vi "FTW-Supervisor-Core-Process.vi"(0 "FTW Supervisor Configuration":string, 11 "error in":errorcluster) -> (15 "error out":errorcluster)   [LabVIEW 2014, in "FTW-Supervisor.lvclass"]
uses:
  FTW-Supervisor.lvclass
  instance/FTW-Actor-Instance.lvclass/FTW-Actor-Instance.ctl
  FTW-Supervisor.lvclass/FTW-Supervisor.ctl
  scheduler/FTW-Scheduler-GetNextJob.vi
  scheduler/FTW-Scheduler-CheckShutdown.vi
  connector/FTW-Supervisor-Connector.lvclass
  instance/FTW-Actor-Instance.lvclass
panel:
  # "Inputs"
  # "Outputs"
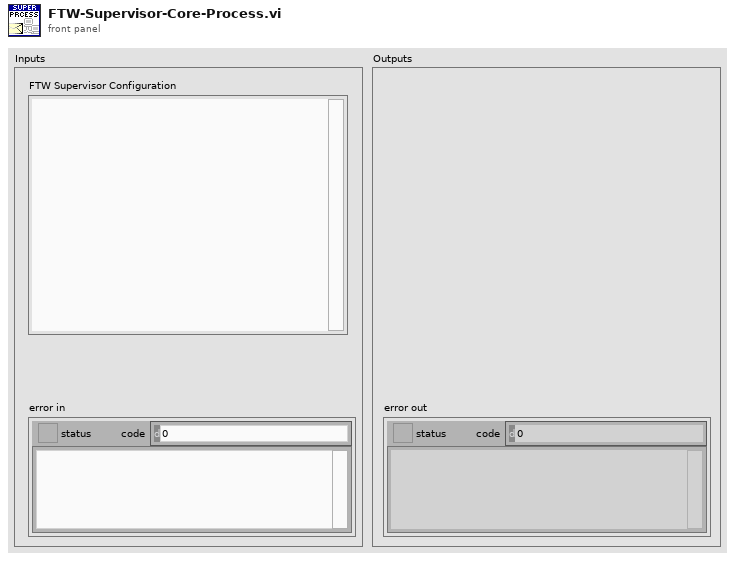
[diagram p1: front panel]
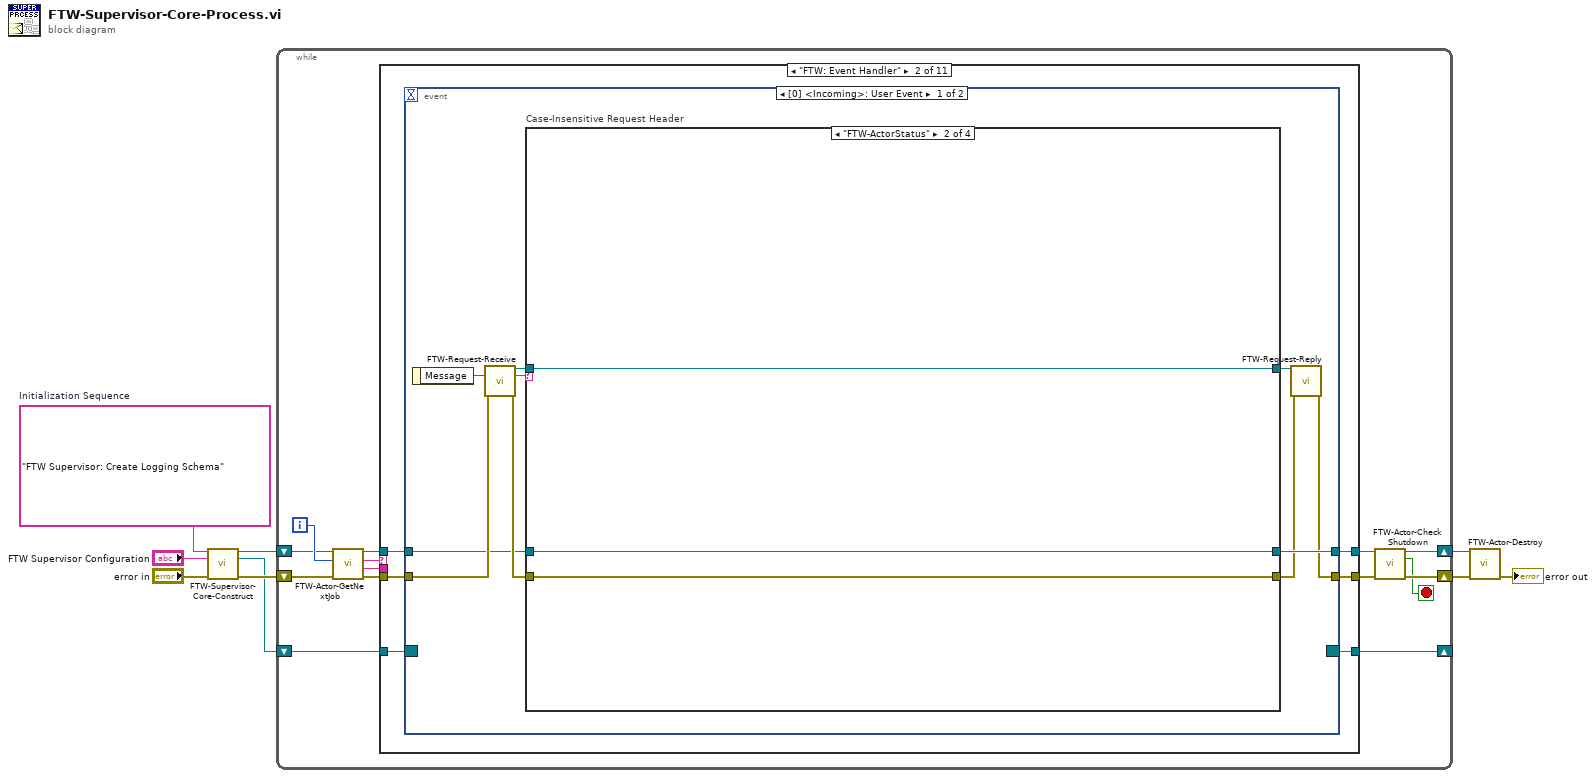
[diagram p0: block diagram]
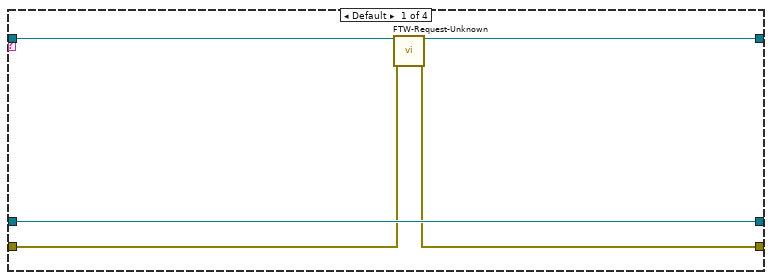
[diagram p3: hidden frame]
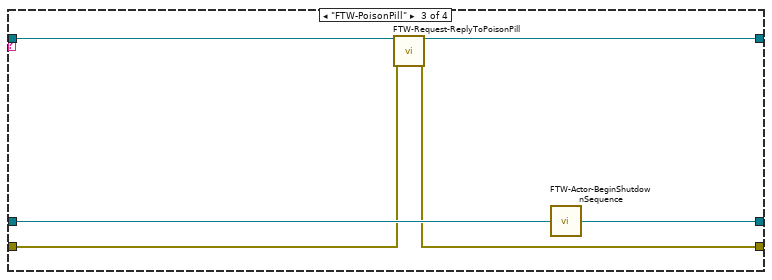
[diagram p4: hidden frame]
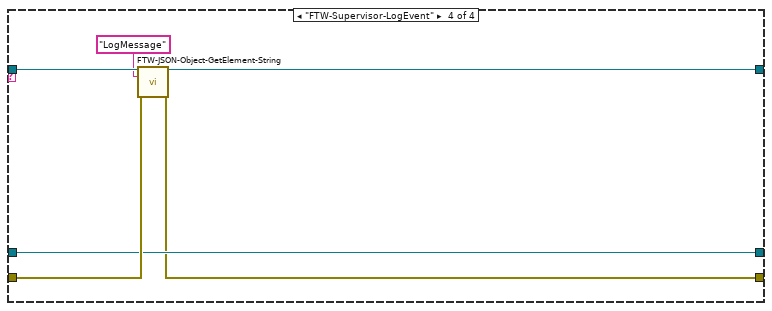
[diagram p5: hidden frame]
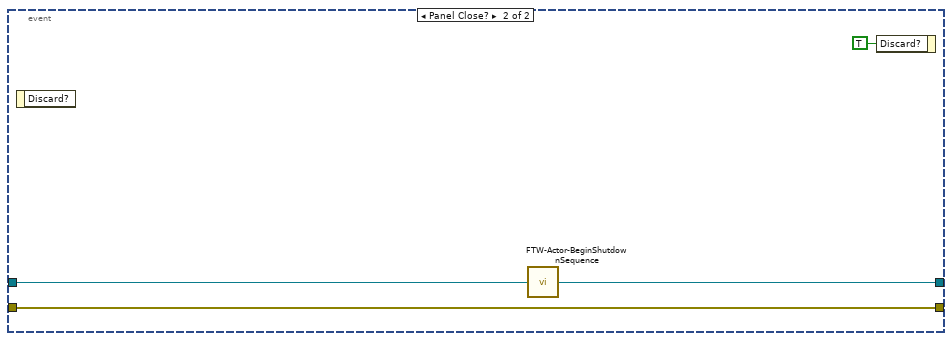
[diagram p6: hidden frame]
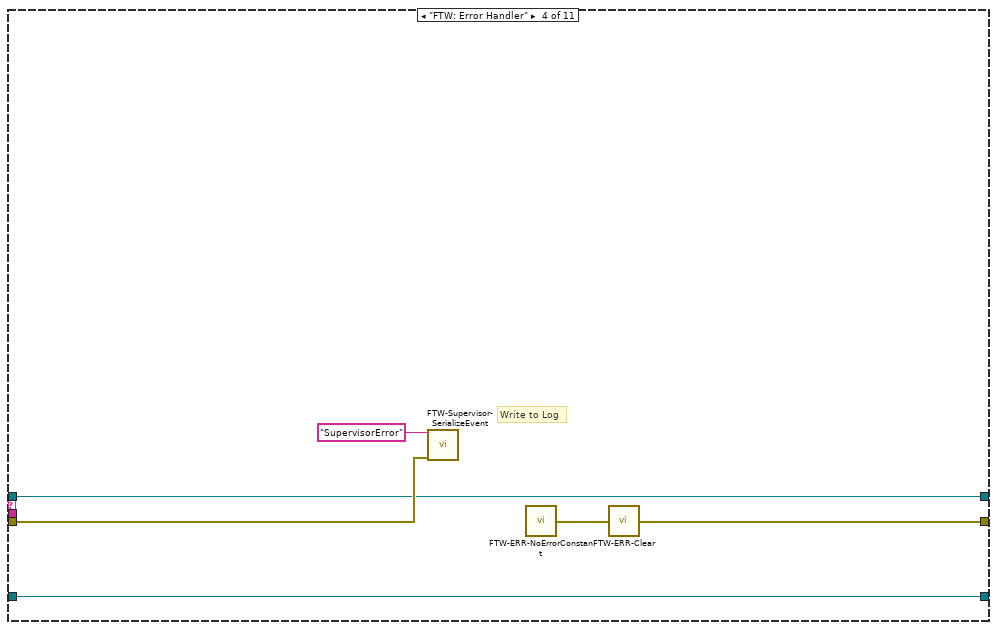
[diagram p8: hidden frame]
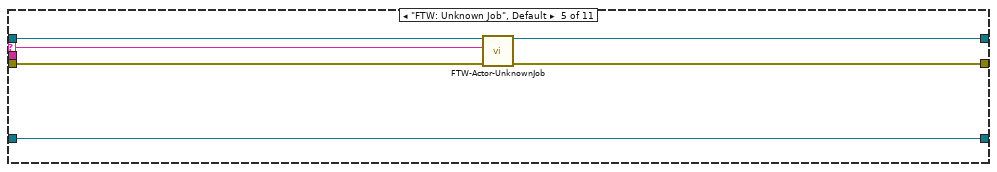
[diagram p9: hidden frame]
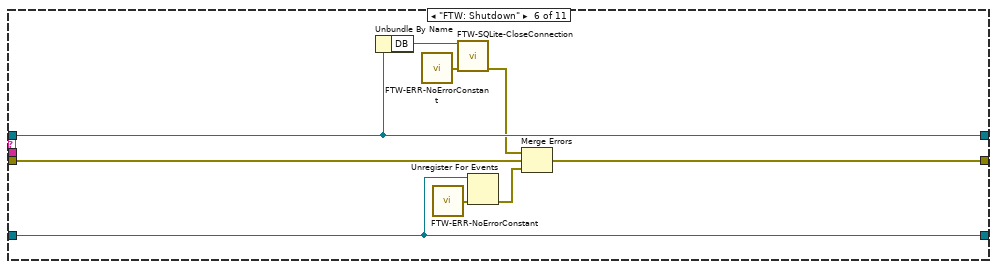
[diagram p10: hidden frame]
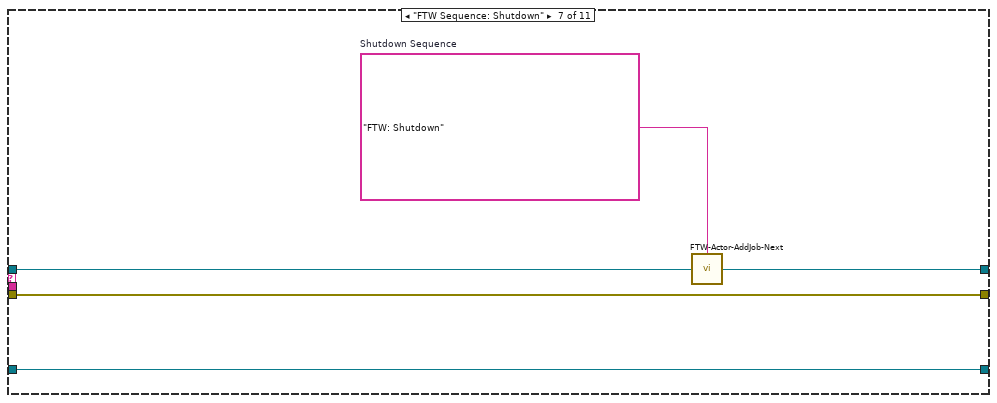
[diagram p11: hidden frame]
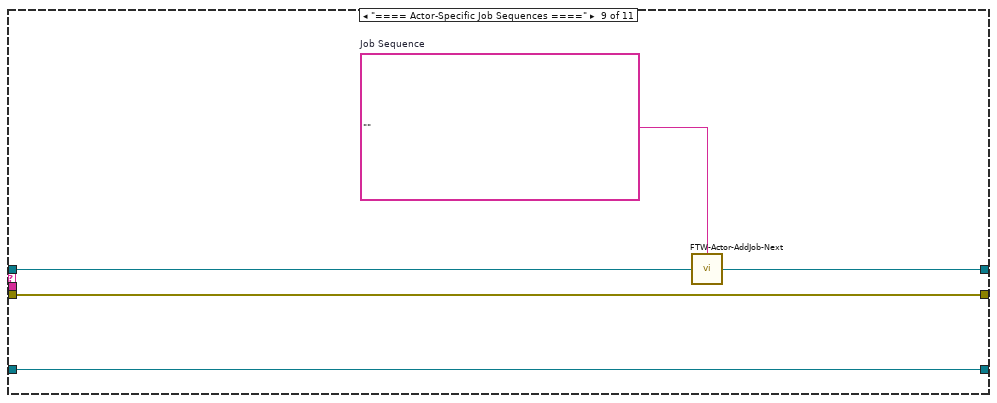
[diagram p13: hidden frame]
diagram:
  w3 = "FTW Supervisor: Create Logging Schema"  # Initialization Sequence
  n1 = call "FTW-Supervisor-Core-Construct.vi"("Initialization Sequence"=w3, "FTW Supervisor Configuration"="FTW Supervisor Configuration", "error in"="error in") -> ("FTW Supervisor"=w6:refnum<class "FTW-Supervisor.lvclass">, "Incoming Request"=w1:refnum<event-registration>, "error out"=w5:errorcluster)  [unwired: 10 in]
  n2 = while {
    shift-right: [w12] -> w8
    shift-left: w5 -> [w21]
    shift-right: [w22] -> _
    shift-left: w1 -> [w23]
    shift-right: [w11] -> w9
    shift-left: w6 -> [w18]
    i -> [w20]
    stop <- w10 stop-if-true
    n3 = call "FTW-Actor-GetNextJob.vi"("error in"=w21, "Jobs Performed"=w20, "FTW Actor Instance"=w18) -> ("error out"=w19:errorcluster, "Job Data"=w15:string, "Job Name"=w16:string, "FTW Actor Instance out"=w17:refnum<class "FTW-Supervisor.lvclass">)  [unwired: 5 in]
    n4 = case shown="\"FTW: Event Handler\"" w16 {
      selector: w16 -> [_ _ _ _ w77 _ _ _ _ _ _]
      tunnel: [w25 w32 w68 w72 w78 w90 w94 w98 w102 w106 w107] -> w13
      tunnel: w19 -> [w25 w31 w68 w73 w76 w87 w94 w98 w102 w106 w107]
      tunnel: w23 -> [w26 w30 w69 w75 w81 w88 w95 w97 w103 w105 w109]
      tunnel: [w26 w29 w69 w75 w81 w88 w95 w97 w103 w105 w109] -> w22
      tunnel: w17 -> [w24 w27 w67 w70 w80 w85 w92 w96 w100 w104 w108]
      tunnel: [w24 w28 w67 w70 w79 w85 w91 w96 w99 w104 w108] -> w14
      tunnel: w15 -> [_ _ _ _ _ _ _ _ _ _ _]
      frame "==== Featherweight Framework Jobs ====" {
      }
      frame "FTW: Event Handler" {
        n5 = event shown="[0] <Incoming>: User Event" {
          selector: w30 -> [_ _]
          dyn-events: [_ _] -> w29
          timeout: _ -> [_ _]
          tunnel: [w35 w65] -> w32
          tunnel: w31 -> [w41 w65]
          tunnel: [w40 w63] -> w28
          tunnel: w27 -> [w39 w64]
          event User Event {
            n6 = event-data() -> ("Message"=w33:refnum<queue>)  [unwired: 1 in]
            n7 = call "FTW-Request-Receive.vi"("MessagePipe"=w33, "error in"=w41) -> ("Request"=w37:refnum<data-value>, "Request Header"=w38:string, "error out"=w42:errorcluster)  [unwired: 11 in]
            n8 = case "Case-Insensitive Request Header" shown="\"FTW-ActorStatus\"" w38 {
              tunnel: [w44 w48 w51 w57] -> w34
              tunnel: w42 -> [w45 w48 w52 w60]
              tunnel: [w47 w50 w55 w58] -> w40
              tunnel: w39 -> [w47 w50 w56 w58]
              tunnel: w37 -> [w46 w49 w54 w62]
              tunnel: [w43 w49 w53 w61] -> w36
              frame Default {
                n9 = call "FTW-Request-Unknown.vi"("Request"=w46, "error in"=w45) -> ("Request out"=w43:refnum<data-value>, "error out"=w44:errorcluster)  [unwired: 12 in]
              }
              frame "FTW-ActorStatus" {
              }
              frame "FTW-PoisonPill" {
                n10 = call "FTW-Request-ReplyToPoisonPill.vi"("Poison Pill Request"=w54, "error in"=w52) -> ("Poison Pill Response"=w53:refnum<data-value>, "error out"=w51:errorcluster)  [unwired: 12 in]
                n11 = call "FTW-Actor-BeginShutdownSequence.vi"("FTW Actor Instance"=w56) -> ("FTW Actor Instance out"=w55:refnum<class "FTW-Supervisor.lvclass">)  [unwired: 3 in]
              }
              frame "FTW-Supervisor-LogEvent" {
                n12 = call "FTW-JSON-Object-GetElement-String.vi"("JSON Object"=w62, "Key"="LogMessage", "error in"=w60) -> ("JSON Object out"=w61:refnum<data-value>, "error out"=w57:errorcluster)  [unwired: 9 in, 2 out]
              }
            }
            n13 = call "FTW-Request-Reply.vi"("Request"=w36, "error in"=w34) -> ("error out"=w35:errorcluster)  [unwired: 13 in]
          }
          event Panel Close? {
            n14 = event-data() -> ()  [unwired: 1 in, 1 out]
            n15 = call "FTW-Actor-BeginShutdownSequence.vi"("FTW Actor Instance"=w64) -> ("FTW Actor Instance out"=w63:refnum<class "FTW-Supervisor.lvclass">)  [unwired: 3 in]
            n16 = event-data("Discard?"=TRUE) -> ()  [unwired: 1 in, 1 out]
          }
        }
      }
      frame "FTW: Failure to Launch" {
      }
      frame "FTW: Error Handler" {
        # "Write to Log"
        n17 = call "FTW-Supervisor-SerializeEvent.vi"("Event Type"="SupervisorError", "Error to Log"=w73) -> ()  [unwired: 13 in, 1 out]
        n18 = call "FTW-ERR-NoErrorConstant.vi"() -> ("no error"=w71:errorcluster)
        n19 = call "FTW-ERR-Clear.vi"("error to snuff"=w71) -> ("no error"=w72:errorcluster)
      }
      frame "FTW: Unknown Job", Default {
        n20 = call-dynamic "FTW-Actor-UnknownJob.vi"("FTW Actor Instance"=w80, "Unknown Job"=w77, "error in"=w76) -> ("FTW Actor Instance out"=w79:refnum<class "FTW-Supervisor.lvclass">, "error out"=w78:errorcluster)  [unwired: 11 in]
      }
      frame "FTW: Shutdown" {
        n21 = Unbundle By Name(w85) -> ("DB"=w86:refnum<data-value>)
        n22 = call "FTW-ERR-NoErrorConstant.vi"() -> ("no error"=w84:errorcluster)
        n23 = call "FTW-ERR-NoErrorConstant.vi"() -> ("no error"=w83:errorcluster)
        n24 = call "FTW-SQLite-CloseConnection.vi"("SQLite Connection"=w86, "error in"=w84) -> ("error out"=w82:errorcluster)  [unwired: 13 in]
        n25 = Unregister For Events(event registration refnum=w88, error in=w83) -> (error out=w89:errorcluster)
        n26 = Merge Errors(w82, w87, w89) -> (w90:errorcluster)
      }
      frame "FTW Sequence: Shutdown" {
        w93 = "FTW: Shutdown"  # Shutdown Sequence
        n27 = call "FTW-Actor-AddJob-Next.vi"("Add Next in Job Queue"=w93, "FTW Actor Instance"=w92) -> ("FTW Actor Instance out"=w91:refnum<class "FTW-Supervisor.lvclass">)  [unwired: 2 in]
      }
      frame "==== Actor-Specific Static Dependencies ====" {
      }
      frame "==== Actor-Specific Job Sequences ====" {
        w101 = ""  # Job Sequence
        n28 = call "FTW-Actor-AddJob-Next.vi"("Add Next in Job Queue"=w101, "FTW Actor Instance"=w100) -> ("FTW Actor Instance out"=w99:refnum<class "FTW-Supervisor.lvclass">)  [unwired: 2 in]
      }
      frame "==== Actor-Specific Jobs ====" {
      }
      frame "FTW Supervisor: Create Logging Schema" {
      }
    }
    n29 = call "FTW-Actor-CheckShutdown.vi"("FTW Actor Instance"=w14, "error in"=w13) -> ("FTW Actor Instance out"=w11:refnum<class "FTW-Supervisor.lvclass">, "Shutdown?"=w10:bool, "error out"=w12:errorcluster)  [unwired: 11 in]
  }
  n30 = call-dynamic "FTW-Actor-Destroy.vi"("FTW Actor Instance"=w9, "error in"=w8) -> ("error out"=→"error out":errorcluster)  [unwired: 13 in]
